vi "AIsFIFO.vi"   [LabVIEW 2010]
uses:
  <vilib>/eio/EIONode/EIONode.xnode
  <vilib>/rvi/DataTransferAndStorage/Container/Common/niFpgaContainerMethod.ctl
  <vilib>/rvi/DataTransferAndStorage/Container/Common/niFpgaTransferTypeControl.ctl
  <vilib>/rvi/interface/RandomDataEmulation/nirviRandomDataFPGAFIFO.vi
  <vilib>/rvi/interface/RandomDataEmulation/niFpgaRandomDataHandleErrors.vi
  <vilib>/rvi/DataTransferAndStorage/Container/XNode/niFpgaContainer.xnode
  <vilib>/rvi/FIFO/Fifo_Types/niFpgaFifoControlLogicControl.ctl
  <vilib>/rvi/DataTransferAndStorage/Container/Common/niFpgaContainerMetaDataKey.ctl
  <vilib>/rvi/DataTransferAndStorage/Container/Common/niFpgaContainerExecOnDevCompGetState.vi
  <vilib>/rvi/FIFO/Fifo_Resource/nirvififoEmulationSetSize.vi
  <vilib>/rvi/DataTransferAndStorage/Container/Common/niFpgaContainerGetUniqueNameForEmu.vi
  <vilib>/rvi/eio/common/nirviEmuReportErrorAndStop.vi
  <vilib>/rvi/DataTransferAndStorage/FIFO/niFpgaPeerToPeerStreamState.ctl
diagram:
  n1 = xnode "FPGA I/O Node"() -> ("Mod1/AI0"=w287, "Mod1/AI1"=w284, "Mod1/AI2"=w281, "Mod1/AI3"=w279, "Mod1/AI4"=w275, "Mod1/AI5"=w272, "Mod1/AI6"=w269, "Mod1/AI7"=w266, "Mod1/AI8"=w263, "Mod1/AI9"=w260, "Mod1/AI10"=w257, "Mod1/AI11"=w254, "Mod1/AI12"=w251, "Mod1/AI13"=w248, "Mod1/AI14"=w245, "Mod1/AI15"=w242, "Mod1/AI16"=w239, "Mod1/AI17"=w236, "Mod1/AI18"=w233, "Mod1/AI19"=w230, "Mod1/AI20"=w227, "Mod1/AI21"=w224, "Mod1/AI22"=w221, "Mod1/AI23"=w218, "Mod1/AI24"=w215, "Mod1/AI25"=w212, "Mod1/AI26"=w209, "Mod1/AI27"=w206, "Mod1/AI28"=w203, "Mod1/AI29"=w200, "Mod1/AI30"=w197, "Mod1/AI31"=w194)  [unwired: 32 in, 32 out]
  n2 = xnode ("FIFO Method Node")("Element"=w287, "Timeout"=10, "FIFO In"=refnum<k21> "FIFO") -> ("FIFO Out"=w285:refnum<k21>)  [unwired: 1 out]
  n3 = xnode ("FIFO Method Node")("Element"=w284, "Timeout"=10, "FIFO In"=w285) -> ("FIFO Out"=w282:refnum<k21>)  [unwired: 1 out]
  n4 = xnode ("FIFO Method Node")("Element"=w281, "Timeout"=10, "FIFO In"=w282) -> ("FIFO Out"=w278:refnum<k21>)  [unwired: 1 out]
  n5 = xnode ("FIFO Method Node")("Element"=w279, "Timeout"=10, "FIFO In"=w278) -> ("FIFO Out"=w276:refnum<k21>)  [unwired: 1 out]
  n6 = xnode ("FIFO Method Node")("Element"=w275, "Timeout"=10, "FIFO In"=w276) -> ("FIFO Out"=w273:refnum<k21>)  [unwired: 1 out]
  n7 = xnode ("FIFO Method Node")("Element"=w272, "Timeout"=10, "FIFO In"=w273) -> ("FIFO Out"=w270:refnum<k21>)  [unwired: 1 out]
  n8 = xnode ("FIFO Method Node")("Element"=w269, "Timeout"=10, "FIFO In"=w270) -> ("FIFO Out"=w267:refnum<k21>)  [unwired: 1 out]
  n9 = xnode ("FIFO Method Node")("Element"=w266, "Timeout"=10, "FIFO In"=w267) -> ("FIFO Out"=w264:refnum<k21>)  [unwired: 1 out]
  n10 = xnode ("FIFO Method Node")("Element"=w263, "Timeout"=10, "FIFO In"=w264) -> ("FIFO Out"=w261:refnum<k21>)  [unwired: 1 out]
  n11 = xnode ("FIFO Method Node")("Element"=w260, "Timeout"=10, "FIFO In"=w261) -> ("FIFO Out"=w258:refnum<k21>)  [unwired: 1 out]
  n12 = xnode ("FIFO Method Node")("Element"=w257, "Timeout"=10, "FIFO In"=w258) -> ("FIFO Out"=w255:refnum<k21>)  [unwired: 1 out]
  n13 = xnode ("FIFO Method Node")("Element"=w254, "Timeout"=10, "FIFO In"=w255) -> ("FIFO Out"=w252:refnum<k21>)  [unwired: 1 out]
  n14 = xnode ("FIFO Method Node")("Element"=w251, "Timeout"=10, "FIFO In"=w252) -> ("FIFO Out"=w249:refnum<k21>)  [unwired: 1 out]
  n15 = xnode ("FIFO Method Node")("Element"=w248, "Timeout"=10, "FIFO In"=w249) -> ("FIFO Out"=w246:refnum<k21>)  [unwired: 1 out]
  n16 = xnode ("FIFO Method Node")("Element"=w245, "Timeout"=10, "FIFO In"=w246) -> ("FIFO Out"=w243:refnum<k21>)  [unwired: 1 out]
  n17 = xnode ("FIFO Method Node")("Element"=w242, "Timeout"=10, "FIFO In"=w243) -> ("FIFO Out"=w240:refnum<k21>)  [unwired: 1 out]
  n18 = xnode ("FIFO Method Node")("Element"=w239, "Timeout"=10, "FIFO In"=w240) -> ("FIFO Out"=w237:refnum<k21>)  [unwired: 1 out]
  n19 = xnode ("FIFO Method Node")("Element"=w236, "Timeout"=10, "FIFO In"=w237) -> ("FIFO Out"=w234:refnum<k21>)  [unwired: 1 out]
  n20 = xnode ("FIFO Method Node")("Element"=w233, "Timeout"=10, "FIFO In"=w234) -> ("FIFO Out"=w231:refnum<k21>)  [unwired: 1 out]
  n21 = xnode ("FIFO Method Node")("Element"=w230, "Timeout"=10, "FIFO In"=w231) -> ("FIFO Out"=w228:refnum<k21>)  [unwired: 1 out]
  n22 = xnode ("FIFO Method Node")("Element"=w227, "Timeout"=10, "FIFO In"=w228) -> ("FIFO Out"=w225:refnum<k21>)  [unwired: 1 out]
  n23 = xnode ("FIFO Method Node")("Element"=w224, "Timeout"=10, "FIFO In"=w225) -> ("FIFO Out"=w222:refnum<k21>)  [unwired: 1 out]
  n24 = xnode ("FIFO Method Node")("Element"=w221, "Timeout"=10, "FIFO In"=w222) -> ("FIFO Out"=w219:refnum<k21>)  [unwired: 1 out]
  n25 = xnode ("FIFO Method Node")("Element"=w218, "Timeout"=10, "FIFO In"=w219) -> ("FIFO Out"=w216:refnum<k21>)  [unwired: 1 out]
  n26 = xnode ("FIFO Method Node")("Element"=w215, "Timeout"=10, "FIFO In"=w216) -> ("FIFO Out"=w213:refnum<k21>)  [unwired: 1 out]
  n27 = xnode ("FIFO Method Node")("Element"=w212, "Timeout"=10, "FIFO In"=w213) -> ("FIFO Out"=w210:refnum<k21>)  [unwired: 1 out]
  n28 = xnode ("FIFO Method Node")("Element"=w209, "Timeout"=10, "FIFO In"=w210) -> ("FIFO Out"=w207:refnum<k21>)  [unwired: 1 out]
  n29 = xnode ("FIFO Method Node")("Element"=w206, "Timeout"=10, "FIFO In"=w207) -> ("FIFO Out"=w204:refnum<k21>)  [unwired: 1 out]
  n30 = xnode ("FIFO Method Node")("Element"=w203, "Timeout"=10, "FIFO In"=w204) -> ("FIFO Out"=w201:refnum<k21>)  [unwired: 1 out]
  n31 = xnode ("FIFO Method Node")("Element"=w200, "Timeout"=10, "FIFO In"=w201) -> ("FIFO Out"=w198:refnum<k21>)  [unwired: 1 out]
  n32 = xnode ("FIFO Method Node")("Element"=w197, "Timeout"=10, "FIFO In"=w198) -> ("FIFO Out"=w195:refnum<k21>)  [unwired: 1 out]
  n33 = xnode ("FIFO Method Node")("Element"=w194, "Timeout"=10, "FIFO In"=w195) -> ("FIFO Out"=w97:refnum<k21>)  [unwired: 1 out]
  n34 = xnode "FPGA I/O Node"() -> ("Mod2/AI0"=w191, "Mod2/AI1"=w188, "Mod2/AI2"=w185, "Mod2/AI3"=w183, "Mod2/AI4"=w179, "Mod2/AI5"=w176, "Mod2/AI6"=w173, "Mod2/AI7"=w170, "Mod2/AI8"=w167, "Mod2/AI9"=w164, "Mod2/AI10"=w161, "Mod2/AI11"=w158, "Mod2/AI12"=w155, "Mod2/AI13"=w152, "Mod2/AI14"=w149, "Mod2/AI15"=w146, "Mod2/AI16"=w143, "Mod2/AI17"=w140, "Mod2/AI18"=w137, "Mod2/AI19"=w134, "Mod2/AI20"=w131, "Mod2/AI21"=w128, "Mod2/AI22"=w125, "Mod2/AI23"=w122, "Mod2/AI24"=w119, "Mod2/AI25"=w116, "Mod2/AI26"=w113, "Mod2/AI27"=w110, "Mod2/AI28"=w107, "Mod2/AI29"=w104, "Mod2/AI30"=w101, "Mod2/AI31"=w98)  [unwired: 32 in, 32 out]
  n35 = xnode ("FIFO Method Node")("Element"=w191, "Timeout"=10, "FIFO In"=w97) -> ("FIFO Out"=w189:refnum<k21>)  [unwired: 1 out]
  n36 = xnode ("FIFO Method Node")("Element"=w188, "Timeout"=10, "FIFO In"=w189) -> ("FIFO Out"=w186:refnum<k21>)  [unwired: 1 out]
  n37 = xnode ("FIFO Method Node")("Element"=w185, "Timeout"=10, "FIFO In"=w186) -> ("FIFO Out"=w182:refnum<k21>)  [unwired: 1 out]
  n38 = xnode ("FIFO Method Node")("Element"=w183, "Timeout"=10, "FIFO In"=w182) -> ("FIFO Out"=w180:refnum<k21>)  [unwired: 1 out]
  n39 = xnode ("FIFO Method Node")("Element"=w179, "Timeout"=10, "FIFO In"=w180) -> ("FIFO Out"=w177:refnum<k21>)  [unwired: 1 out]
  n40 = xnode ("FIFO Method Node")("Element"=w176, "Timeout"=10, "FIFO In"=w177) -> ("FIFO Out"=w174:refnum<k21>)  [unwired: 1 out]
  n41 = xnode ("FIFO Method Node")("Element"=w173, "Timeout"=10, "FIFO In"=w174) -> ("FIFO Out"=w171:refnum<k21>)  [unwired: 1 out]
  n42 = xnode ("FIFO Method Node")("Element"=w170, "Timeout"=10, "FIFO In"=w171) -> ("FIFO Out"=w168:refnum<k21>)  [unwired: 1 out]
  n43 = xnode ("FIFO Method Node")("Element"=w167, "Timeout"=10, "FIFO In"=w168) -> ("FIFO Out"=w165:refnum<k21>)  [unwired: 1 out]
  n44 = xnode ("FIFO Method Node")("Element"=w164, "Timeout"=10, "FIFO In"=w165) -> ("FIFO Out"=w162:refnum<k21>)  [unwired: 1 out]
  n45 = xnode ("FIFO Method Node")("Element"=w161, "Timeout"=10, "FIFO In"=w162) -> ("FIFO Out"=w159:refnum<k21>)  [unwired: 1 out]
  n46 = xnode ("FIFO Method Node")("Element"=w158, "Timeout"=10, "FIFO In"=w159) -> ("FIFO Out"=w156:refnum<k21>)  [unwired: 1 out]
  n47 = xnode ("FIFO Method Node")("Element"=w155, "Timeout"=10, "FIFO In"=w156) -> ("FIFO Out"=w153:refnum<k21>)  [unwired: 1 out]
  n48 = xnode ("FIFO Method Node")("Element"=w152, "Timeout"=10, "FIFO In"=w153) -> ("FIFO Out"=w150:refnum<k21>)  [unwired: 1 out]
  n49 = xnode ("FIFO Method Node")("Element"=w149, "Timeout"=10, "FIFO In"=w150) -> ("FIFO Out"=w147:refnum<k21>)  [unwired: 1 out]
  n50 = xnode ("FIFO Method Node")("Element"=w146, "Timeout"=10, "FIFO In"=w147) -> ("FIFO Out"=w144:refnum<k21>)  [unwired: 1 out]
  n51 = xnode ("FIFO Method Node")("Element"=w143, "Timeout"=10, "FIFO In"=w144) -> ("FIFO Out"=w141:refnum<k21>)  [unwired: 1 out]
  n52 = xnode ("FIFO Method Node")("Element"=w140, "Timeout"=10, "FIFO In"=w141) -> ("FIFO Out"=w138:refnum<k21>)  [unwired: 1 out]
  n53 = xnode ("FIFO Method Node")("Element"=w137, "Timeout"=10, "FIFO In"=w138) -> ("FIFO Out"=w135:refnum<k21>)  [unwired: 1 out]
  n54 = xnode ("FIFO Method Node")("Element"=w134, "Timeout"=10, "FIFO In"=w135) -> ("FIFO Out"=w132:refnum<k21>)  [unwired: 1 out]
  n55 = xnode ("FIFO Method Node")("Element"=w131, "Timeout"=10, "FIFO In"=w132) -> ("FIFO Out"=w129:refnum<k21>)  [unwired: 1 out]
  n56 = xnode ("FIFO Method Node")("Element"=w128, "Timeout"=10, "FIFO In"=w129) -> ("FIFO Out"=w126:refnum<k21>)  [unwired: 1 out]
  n57 = xnode ("FIFO Method Node")("Element"=w125, "Timeout"=10, "FIFO In"=w126) -> ("FIFO Out"=w123:refnum<k21>)  [unwired: 1 out]
  n58 = xnode ("FIFO Method Node")("Element"=w122, "Timeout"=10, "FIFO In"=w123) -> ("FIFO Out"=w120:refnum<k21>)  [unwired: 1 out]
  n59 = xnode ("FIFO Method Node")("Element"=w119, "Timeout"=10, "FIFO In"=w120) -> ("FIFO Out"=w117:refnum<k21>)  [unwired: 1 out]
  n60 = xnode ("FIFO Method Node")("Element"=w116, "Timeout"=10, "FIFO In"=w117) -> ("FIFO Out"=w114:refnum<k21>)  [unwired: 1 out]
  n61 = xnode ("FIFO Method Node")("Element"=w113, "Timeout"=10, "FIFO In"=w114) -> ("FIFO Out"=w111:refnum<k21>)  [unwired: 1 out]
  n62 = xnode ("FIFO Method Node")("Element"=w110, "Timeout"=10, "FIFO In"=w111) -> ("FIFO Out"=w108:refnum<k21>)  [unwired: 1 out]
  n63 = xnode ("FIFO Method Node")("Element"=w107, "Timeout"=10, "FIFO In"=w108) -> ("FIFO Out"=w105:refnum<k21>)  [unwired: 1 out]
  n64 = xnode ("FIFO Method Node")("Element"=w104, "Timeout"=10, "FIFO In"=w105) -> ("FIFO Out"=w102:refnum<k21>)  [unwired: 1 out]
  n65 = xnode ("FIFO Method Node")("Element"=w101, "Timeout"=10, "FIFO In"=w102) -> ("FIFO Out"=w99:refnum<k21>)  [unwired: 1 out]
  n66 = xnode ("FIFO Method Node")("Element"=w98, "Timeout"=10, "FIFO In"=w99) -> ("FIFO Out"=w1:refnum<k21>)  [unwired: 1 out]
  n67 = xnode "FPGA I/O Node"() -> ("Mod3/AI0"=w95, "Mod3/AI1"=w92, "Mod3/AI2"=w89, "Mod3/AI3"=w87, "Mod3/AI4"=w83, "Mod3/AI5"=w80, "Mod3/AI6"=w77, "Mod3/AI7"=w74, "Mod3/AI8"=w71, "Mod3/AI9"=w68, "Mod3/AI10"=w65, "Mod3/AI11"=w62, "Mod3/AI12"=w59, "Mod3/AI13"=w56, "Mod3/AI14"=w53, "Mod3/AI15"=w50, "Mod3/AI16"=w47, "Mod3/AI17"=w44, "Mod3/AI18"=w41, "Mod3/AI19"=w38, "Mod3/AI20"=w35, "Mod3/AI21"=w32, "Mod3/AI22"=w29, "Mod3/AI23"=w26, "Mod3/AI24"=w23, "Mod3/AI25"=w20, "Mod3/AI26"=w17, "Mod3/AI27"=w14, "Mod3/AI28"=w11, "Mod3/AI29"=w8, "Mod3/AI30"=w5, "Mod3/AI31"=w2)  [unwired: 32 in, 32 out]
  n68 = xnode ("FIFO Method Node")("Element"=w95, "Timeout"=10, "FIFO In"=w1) -> ("FIFO Out"=w93:refnum<k21>)  [unwired: 1 out]
  n69 = xnode ("FIFO Method Node")("Element"=w92, "Timeout"=10, "FIFO In"=w93) -> ("FIFO Out"=w90:refnum<k21>)  [unwired: 1 out]
  n70 = xnode ("FIFO Method Node")("Element"=w89, "Timeout"=10, "FIFO In"=w90) -> ("FIFO Out"=w86:refnum<k21>)  [unwired: 1 out]
  n71 = xnode ("FIFO Method Node")("Element"=w87, "Timeout"=10, "FIFO In"=w86) -> ("FIFO Out"=w84:refnum<k21>)  [unwired: 1 out]
  n72 = xnode ("FIFO Method Node")("Element"=w83, "Timeout"=10, "FIFO In"=w84) -> ("FIFO Out"=w81:refnum<k21>)  [unwired: 1 out]
  n73 = xnode ("FIFO Method Node")("Element"=w80, "Timeout"=10, "FIFO In"=w81) -> ("FIFO Out"=w78:refnum<k21>)  [unwired: 1 out]
  n74 = xnode ("FIFO Method Node")("Element"=w77, "Timeout"=10, "FIFO In"=w78) -> ("FIFO Out"=w75:refnum<k21>)  [unwired: 1 out]
  n75 = xnode ("FIFO Method Node")("Element"=w74, "Timeout"=10, "FIFO In"=w75) -> ("FIFO Out"=w72:refnum<k21>)  [unwired: 1 out]
  n76 = xnode ("FIFO Method Node")("Element"=w71, "Timeout"=10, "FIFO In"=w72) -> ("FIFO Out"=w69:refnum<k21>)  [unwired: 1 out]
  n77 = xnode ("FIFO Method Node")("Element"=w68, "Timeout"=10, "FIFO In"=w69) -> ("FIFO Out"=w66:refnum<k21>)  [unwired: 1 out]
  n78 = xnode ("FIFO Method Node")("Element"=w65, "Timeout"=10, "FIFO In"=w66) -> ("FIFO Out"=w63:refnum<k21>)  [unwired: 1 out]
  n79 = xnode ("FIFO Method Node")("Element"=w62, "Timeout"=10, "FIFO In"=w63) -> ("FIFO Out"=w60:refnum<k21>)  [unwired: 1 out]
  n80 = xnode ("FIFO Method Node")("Element"=w59, "Timeout"=10, "FIFO In"=w60) -> ("FIFO Out"=w57:refnum<k21>)  [unwired: 1 out]
  n81 = xnode ("FIFO Method Node")("Element"=w56, "Timeout"=10, "FIFO In"=w57) -> ("FIFO Out"=w54:refnum<k21>)  [unwired: 1 out]
  n82 = xnode ("FIFO Method Node")("Element"=w53, "Timeout"=10, "FIFO In"=w54) -> ("FIFO Out"=w51:refnum<k21>)  [unwired: 1 out]
  n83 = xnode ("FIFO Method Node")("Element"=w50, "Timeout"=10, "FIFO In"=w51) -> ("FIFO Out"=w48:refnum<k21>)  [unwired: 1 out]
  n84 = xnode ("FIFO Method Node")("Element"=w47, "Timeout"=10, "FIFO In"=w48) -> ("FIFO Out"=w45:refnum<k21>)  [unwired: 1 out]
  n85 = xnode ("FIFO Method Node")("Element"=w44, "Timeout"=10, "FIFO In"=w45) -> ("FIFO Out"=w42:refnum<k21>)  [unwired: 1 out]
  n86 = xnode ("FIFO Method Node")("Element"=w41, "Timeout"=10, "FIFO In"=w42) -> ("FIFO Out"=w39:refnum<k21>)  [unwired: 1 out]
  n87 = xnode ("FIFO Method Node")("Element"=w38, "Timeout"=10, "FIFO In"=w39) -> ("FIFO Out"=w36:refnum<k21>)  [unwired: 1 out]
  n88 = xnode ("FIFO Method Node")("Element"=w35, "Timeout"=10, "FIFO In"=w36) -> ("FIFO Out"=w33:refnum<k21>)  [unwired: 1 out]
  n89 = xnode ("FIFO Method Node")("Element"=w32, "Timeout"=10, "FIFO In"=w33) -> ("FIFO Out"=w30:refnum<k21>)  [unwired: 1 out]
  n90 = xnode ("FIFO Method Node")("Element"=w29, "Timeout"=10, "FIFO In"=w30) -> ("FIFO Out"=w27:refnum<k21>)  [unwired: 1 out]
  n91 = xnode ("FIFO Method Node")("Element"=w26, "Timeout"=10, "FIFO In"=w27) -> ("FIFO Out"=w24:refnum<k21>)  [unwired: 1 out]
  n92 = xnode ("FIFO Method Node")("Element"=w23, "Timeout"=10, "FIFO In"=w24) -> ("FIFO Out"=w21:refnum<k21>)  [unwired: 1 out]
  n93 = xnode ("FIFO Method Node")("Element"=w20, "Timeout"=10, "FIFO In"=w21) -> ("FIFO Out"=w18:refnum<k21>)  [unwired: 1 out]
  n94 = xnode ("FIFO Method Node")("Element"=w17, "Timeout"=10, "FIFO In"=w18) -> ("FIFO Out"=w15:refnum<k21>)  [unwired: 1 out]
  n95 = xnode ("FIFO Method Node")("Element"=w14, "Timeout"=10, "FIFO In"=w15) -> ("FIFO Out"=w12:refnum<k21>)  [unwired: 1 out]
  n96 = xnode ("FIFO Method Node")("Element"=w11, "Timeout"=10, "FIFO In"=w12) -> ("FIFO Out"=w9:refnum<k21>)  [unwired: 1 out]
  n97 = xnode ("FIFO Method Node")("Element"=w8, "Timeout"=10, "FIFO In"=w9) -> ("FIFO Out"=w6:refnum<k21>)  [unwired: 1 out]
  n98 = xnode ("FIFO Method Node")("Element"=w5, "Timeout"=10, "FIFO In"=w6) -> ("FIFO Out"=w3:refnum<k21>)  [unwired: 1 out]
  n99 = xnode ("FIFO Method Node")("Element"=w2, "Timeout"=10, "FIFO In"=w3) -> ()  [unwired: 2 out]
